vi "Wrap Delta.vi"(9 "B":refnum<class "Vector 2D.lvclass">, 10 "A":refnum<class "Vector 2D.lvclass">, 11 "Camera in":refnum<class "Camera.lvclass">) -> (3 "Wrapped Delta":refnum<class "Vector 2D.lvclass">)   [LabVIEW 2021, in "Camera.lvclass"]
uses:
  Camera.lvclass
  Re-use Libraries/Vector 2D/Vector 2D.lvclass
  Camera.lvclass/Camera.ctl
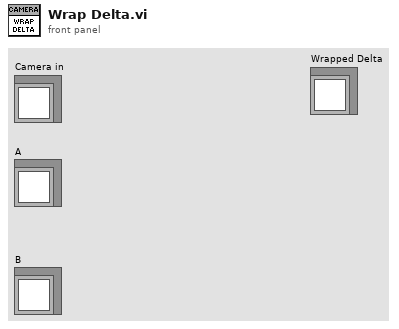
[diagram p1: front panel]
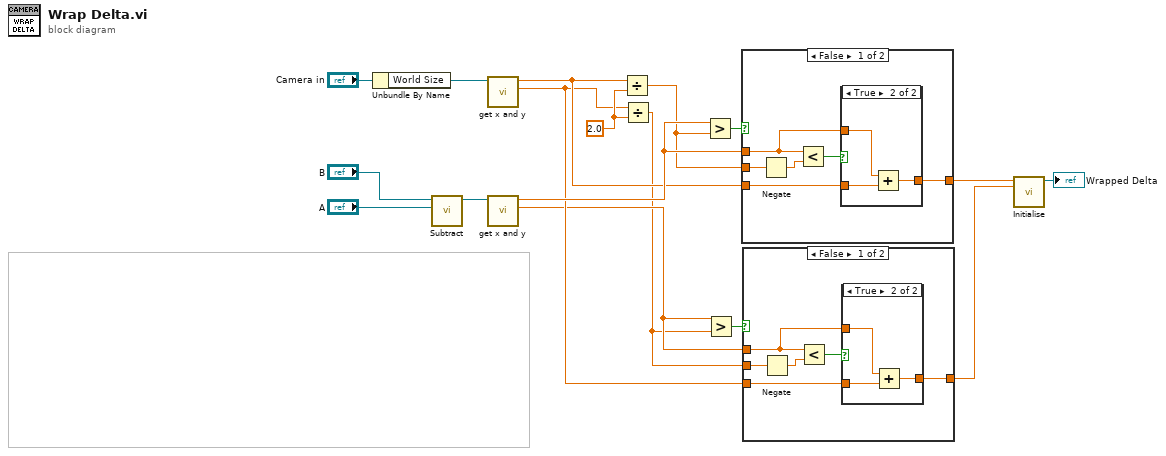
[diagram p0: block diagram]
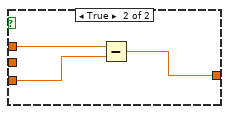
[diagram p3: hidden frame]
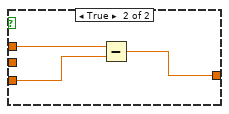
[diagram p5: hidden frame]
diagram:
  w11 = sgl 2.0 ("y")
  n1 = Unbundle By Name("Camera in") -> ("World Size"=w12:refnum<class "Vector 2D.lvclass">)
  n2 = call "Subtract.vi"("B"="A", "A"="B") -> ("A-B"=w13:refnum<class "Vector 2D.lvclass">)  [unwired: 9 in]
  n3 = call "get x and y.vi"("Vector 2D in"=w12) -> ("y"=w5:sgl, "x"=w8:sgl)  [unwired: 9 in]
  n4 = call "get x and y.vi"("Vector 2D in"=w13) -> ("y"=w4:sgl, "x"=w9:sgl)  [unwired: 9 in]
  n5 = Divide(x=w8, y=w11) -> (x/y=w2:sgl)
  n6 = Divide(x=w5, y=w11) -> (x/y=w1:sgl)
  n7 = Greater?(x=w9, y=w2) -> (0:w10:bool)
  n8 = Greater?(x=w4, y=w1) -> (0:w6:bool)
  n9 = case shown="False" w10 {
    tunnel: w9 -> [w21 w30]
    tunnel: w8 -> [w19 w29]
    tunnel: [w20 w28] -> w7
    tunnel: w2 -> [w18 _]
    frame False {
      n10 = Negate(x=w18) -> (-x=w23:sgl)
      n11 = Less?(x=w21, y=w23) -> (x < y?=w22:bool)
      n12 = case shown="True" w22 {
        tunnel: w21 -> [w24 w27]
        tunnel: [w24 w26] -> w20
        tunnel: w19 -> [_ w25]
        frame False {
        }
        frame True {
          n13 = Add(x=w27, y=w25) -> (x+y=w26:sgl)
        }
      }
    }
    frame True {
      n14 = Subtract(x=w30, y=w29) -> (x-y=w28:sgl)
    }
  }
  n15 = case shown="False" w6 {
    tunnel: w4 -> [w34 w43]
    tunnel: w5 -> [w32 w42]
    tunnel: [w33 w41] -> w3
    tunnel: w1 -> [w31 _]
    frame False {
      n16 = Negate(x=w31) -> (-x=w36:sgl)
      n17 = Less?(x=w34, y=w36) -> (x < y?=w35:bool)
      n18 = case shown="True" w35 {
        tunnel: w34 -> [w37 w40]
        tunnel: [w37 w39] -> w33
        tunnel: w32 -> [_ w38]
        frame False {
        }
        frame True {
          n19 = Add(x=w40, y=w38) -> (x+y=w39:sgl)
        }
      }
    }
    frame True {
      n20 = Subtract(x=w43, y=w42) -> (x-y=w41:sgl)
    }
  }
  n21 = call "Initialise.vi"("y"=w3, "x"=w7) -> ("Vector 2D out"=→"Wrapped Delta":refnum<class "Vector 2D.lvclass">)  [unwired: 9 in]
